vi "RFID_Table_v2.vi"(7 "RFID":string, 8 "error in (no error)":errorcluster, 11 "Ref In":T1={"MS SQL Connection"=refnum, "UDL File"=path "", "Time"="", "DCODE"="", "WIP+1"=0, "MC No?"=0, "POKAYOKE?"=FALSE, "Expected Result"="", "Result [Status]"="", "Clock"=0.0, "RFID"="", "WIP Queue"=refnum, "TS Parameter"={"ProfitCenterCode"="", "LineCode"="", "WorkOrderNumber"="", "Model"="", "Model_with_Prefix"="", "VendorCode"="", "SetParameterDateCode"="", "PokaYoke"=0, "Target"=1, "Live_DateCode"="", "CustomerPartNumber"="", "Hand"="", "Ent_Stamp"=timestamp(0 s since 1904-01-01), "sBarcode"=FALSE, "FCA"=0, "STS_CD"=0.0}, "Data_Queue"=[], "RFID Serial No."=""} {"TS Parameter"."FCA" format="%01d"; "TS Parameter"."Target" min=1 max=100000; "TS Parameter"."PokaYoke" min=0 max=1}) -> (0 "error out":errorcluster)   [LabVIEW 2020]
uses:
  Controls/TD SQL.ctl
  <vilib>/addons/database/Connection.llb/Conn ObjectReference.ctl
  Controls/WIP_State.ctl
  Controls/TS_Parameter.ctl
  <vilib>/Utility/miscctls.llb/LVRowAndColumnUnsignedTypeDef.ctl
  <vilib>/addons/database/NI_Database_API.lvlib
panel:
  in  "Exit":bool
  in  "RFID Details":i32(listbox)
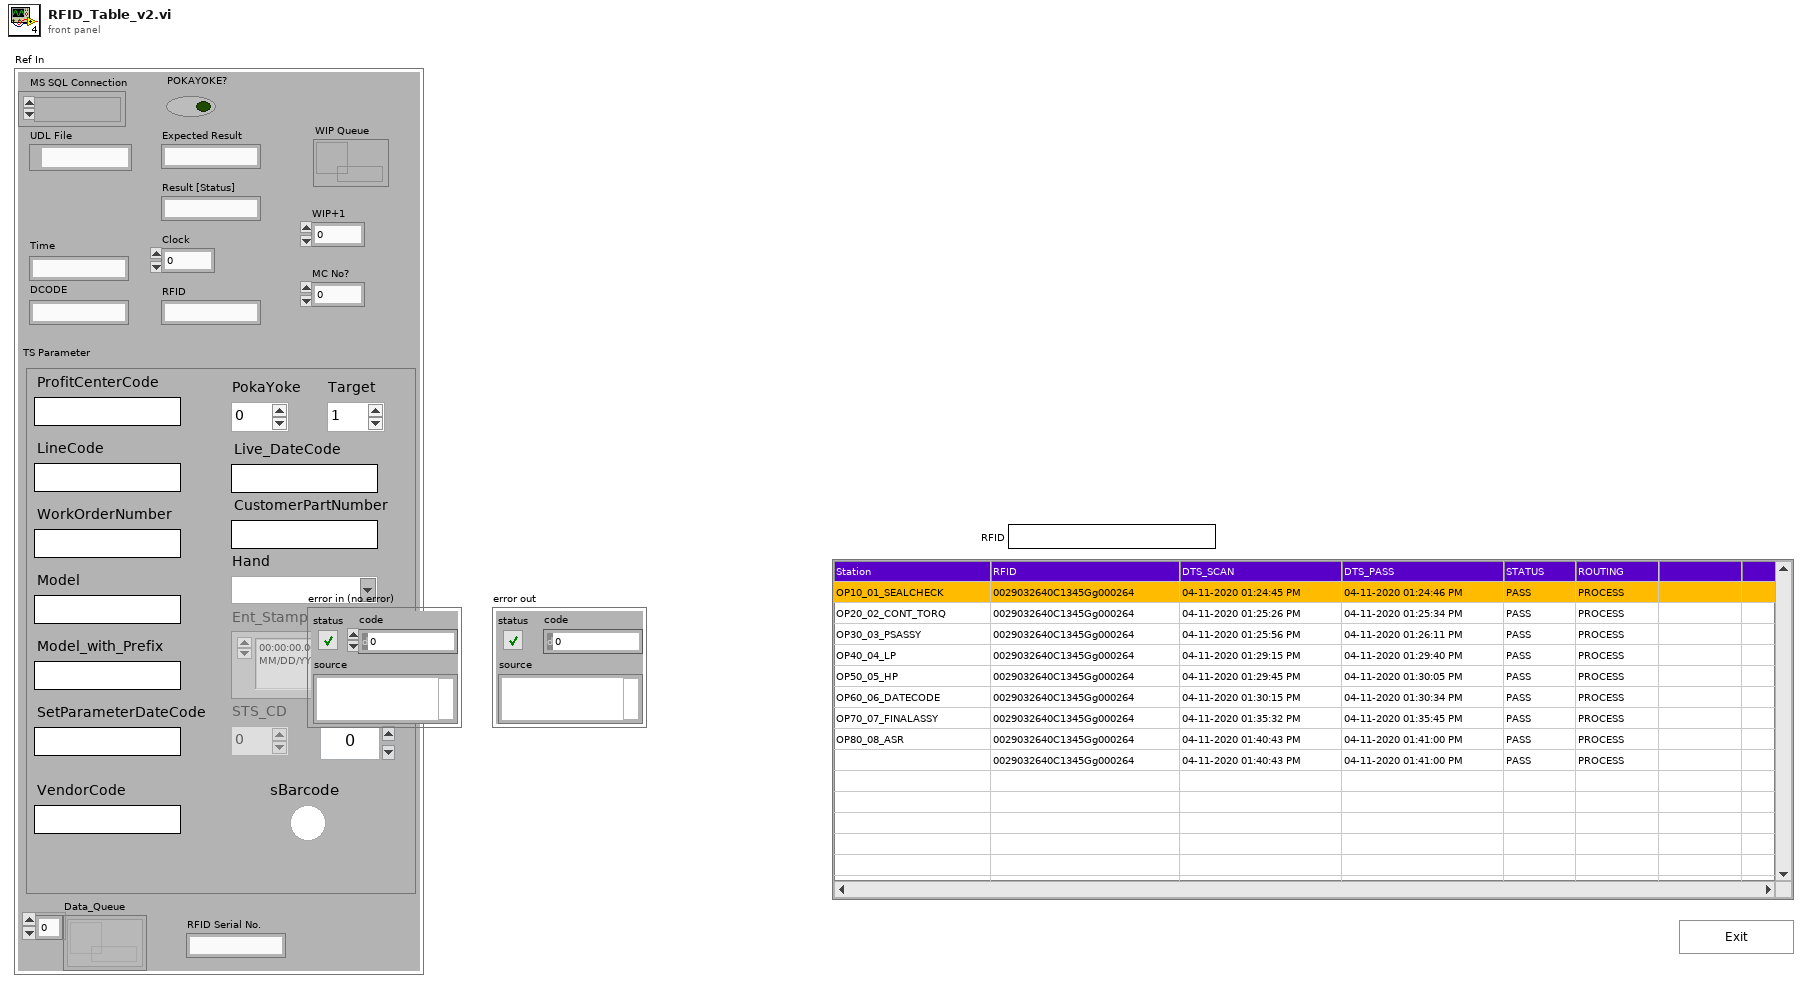
[diagram p1: front panel]
types:
  T1 = typedef "TD SQL.ctl" = cluster{"MS SQL Connection":T2, "UDL File":path, "Time":string, "DCODE":string, "WIP+1":i64, "MC No?":i32, "POKAYOKE?":bool, "Expected Result":string, "Result [Status]":string, "Clock":dbl, "RFID":string, "WIP Queue":refnum<queue>, "TS Parameter":T3, "Data_Queue":refnum<queue>[], "RFID Serial No.":string}
  T2 = typedef "NI_Database_API.lvlib/Conn ObjectReference.ctl" = refnum<k1>
  T3 = typedef "TS_Parameter.ctl" = cluster{"ProfitCenterCode":string, "LineCode":string, "WorkOrderNumber":string, "Model":string, "Model_with_Prefix":string, "VendorCode":string, "SetParameterDateCode":string, "PokaYoke":i32, "Target":i32, "Live_DateCode":string, "CustomerPartNumber":string, "Hand":string, "Ent_Stamp":timestamp, "sBarcode":bool, "FCA":i32, "STS_CD":dbl}
  T4 = typedef "LVRowAndColumnUnsignedTypeDef.ctl" = cluster{"Row":u32, "Column":u32}
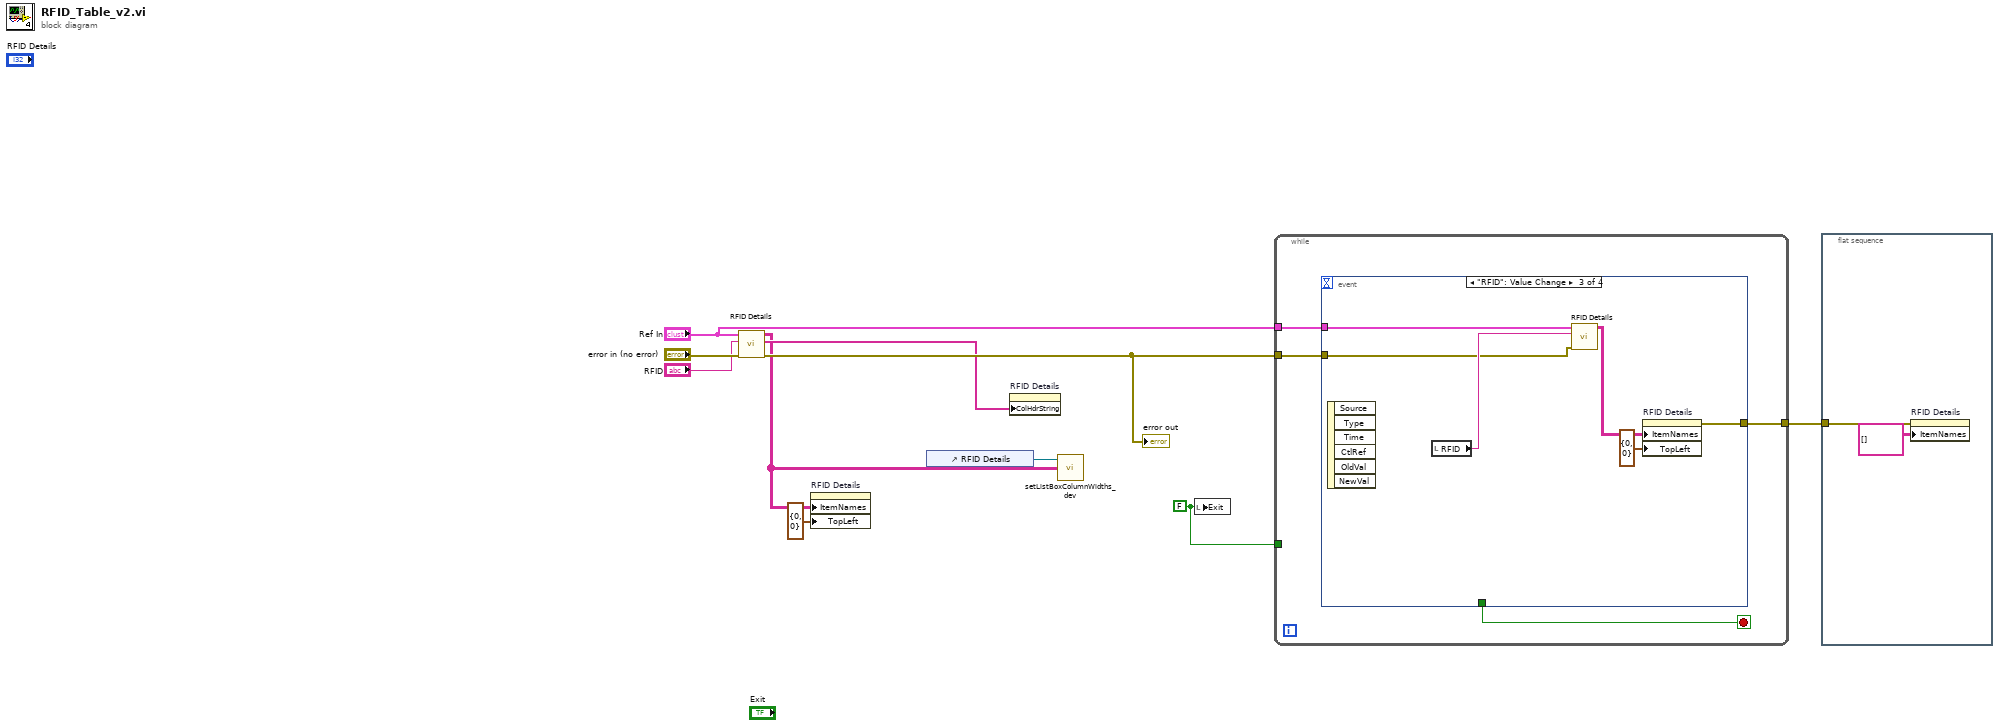
[diagram p0: block diagram]
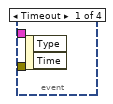
[diagram p2: hidden frame]
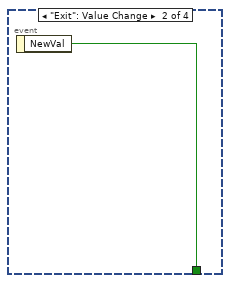
[diagram p3: hidden frame]
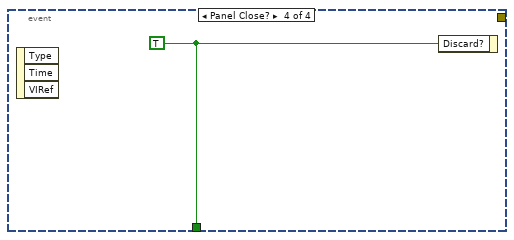
[diagram p4: hidden frame]
diagram:
  w6 = FALSE ("Exit")
  n1 = call "RFID Details.vi"("error in (no error)"="error in (no error)", "RFID"="RFID", "Ref In"="Ref In") -> ("error out"=w8:errorcluster, "Header"=w7:string[], "Data"=w2:string[][])  [unwired: 6 in]
  "error out" <- w8
  n2 = property on="RFID Details" class="MCListbox (strict)"("ItemNames"=w2, "TopLeft"=T4 {"Row"=0, "Column"=0} ("Top Left Visible Cell")) -> ()  [unwired: 2 in, 2 out]
  n3 = control-ref of="RFID Details"() -> (w3:refnum<vi>)
  n4 = property on="RFID Details" class="MCListbox (strict)"("ColHdrString"=w7) -> ()  [unwired: 2 in, 2 out]
  n5 = call "setListBoxColumnWidths_dev.vi"("table data"=w2, "MCListbox Refnum"=w3) -> ()  [unwired: 1 in]
  n6 = local write "Exit"(w6) -> ()
  n7 = while {
    tunnel: w8 -> [w12]
    tunnel: w6 -> [_]
    tunnel: "Ref In" -> [w13]
    tunnel: [w11] -> w1
    stop <- w14 stop-if-true
    n8 = event shown="[2] \"RFID\": Value Change" {
      selector: _ -> [_ _ _ _]
      dyn-events: _ -> [_ _ _ _]
      timeout: _ -> [_ _ _ _]
      tunnel: [_ w15 _ w22] -> w14
      tunnel: w13 -> [_ _ w21 _]
      tunnel: w12 -> [_ _ w19 _]
      tunnel: [_ _ w16 _] -> w11
      event Timeout {
        n9 = event-data() -> ()  [unwired: 1 in, 2 out]
      }
      event "Exit": Value Change {
        n10 = event-data() -> ("NewVal"=w15:bool)  [unwired: 1 in]
      }
      event "RFID": Value Change {
        n11 = event-data() -> ()  [unwired: 1 in, 6 out]
        n12 = local read "RFID"() -> (w20:string)
        n13 = call "RFID Details.vi"("error in (no error)"=w19, "RFID"=w20, "Ref In"=w21) -> ("Data"=w18:string[][])  [unwired: 6 in, 2 out]
        n14 = property on="RFID Details" class="MCListbox (strict)"("ItemNames"=w18, "TopLeft"=T4 {"Row"=0, "Column"=0} ("Top Left Visible Cell")) -> (error out=w16:errorcluster)  [unwired: 2 in, 1 out]
      }
      event Panel Close? {
        w22 = TRUE ("Discard?")
        n15 = event-data() -> ()  [unwired: 1 in, 3 out]
        n16 = event-data("Discard?"=w22) -> ()  [unwired: 1 in, 1 out]
      }
    }
  }
  n17 = flat-sequence {
    tunnel: w1 -> [w24]
    frame #0 {
      n18 = property on="RFID Details" class="MCListbox (strict)"(error in=w24, "ItemNames"=string[][] [] ("Item Names")) -> ()  [unwired: 1 in, 2 out]
    }
  }
